vi "Example2.vi"() -> ()   [LabVIEW 2019]
panel:
  out "C":dbl
  in  "B":dbl
  in  "A":dbl
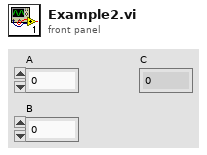
[diagram p1: front panel]
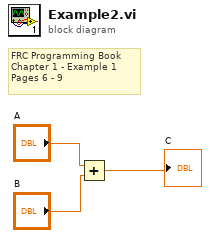
[diagram p0: block diagram]
diagram:
  # "FRC Programming Book\nChapter 1 - Example 1\nPages 6 - 9"
  n1 = Add(x="A", y="B") -> (x+y=→"C":dbl)
